vi "Get PublicEventRegistration.vi"(8 "error in (no error)":errorcluster, 11 "SMO":refnum<class "SMO.lvclass">) -> (0 "error out":errorcluster, 2 "SMO Public Events":refnum<event-registration>, 3 "SMO out":refnum<class "SMO.lvclass">)   [LabVIEW 2021, in "smo.lvlib" / "SMO.lvclass"]
doc: "This method has been deprecated. To achieve the same result, you should use the GetPublicEvents method and register for the events in the process."
uses:
  SMO.lvclass
  SMO.lvclass/SMO.ctl
  Typedefs/Public Events.ctl
  Typedefs/SMOState --Enum.ctl
  Typedefs/Reserve State--Enum.ctl
panel:
  # "For instructions on how to use the JKI State Machine Objects, examples and video tutorials, visit:\nhttp://jki.net/state-machine-objects/\n\nJKI State Machine Objects™\nhttp://jki.net/state-machine-objects/\nCopyright (C) 2005-2015, JKI <info@jki.net>\nALL RIGHTS RESERVED"
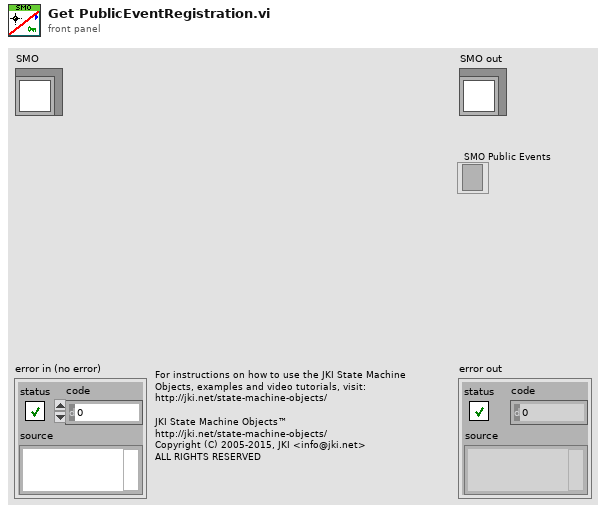
[diagram p1: front panel]
types:
  T1 = typedef "smo.lvlib/SMO.lvclass/Public Events.ctl" = cluster{"Error":refnum<user-event>, "State":refnum<user-event>, "Reserve State":refnum<user-event>}
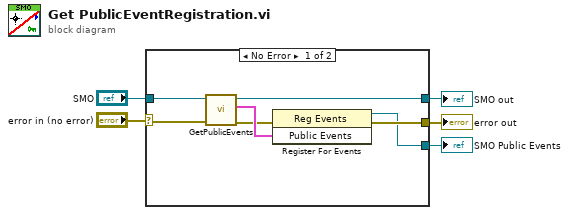
[diagram p0: block diagram]
diagram:
  n1 = case shown="No Error" "error in (no error)" {
    selector: "error in (no error)" -> [w7 w14]
    tunnel: [w12 w14] -> w2
    tunnel: [w8 w13] -> w3
    tunnel: "SMO" -> [w10 w13]
    tunnel: [w11 _] -> w1
    frame No Error {
      n2 = call "GetPublicEvents.vi"("error in (no error)"=w7, "SMO"=w10) -> ("error out"=w6:errorcluster, "Public Events"=w9:T1, "SMO out"=w8:refnum<class "SMO.lvclass">)  [unwired: 7 in]
      n3 = register-events(error in=w6, w9) -> (reference out=w11:refnum<event-registration>, error out=w12:errorcluster)  [unwired: 1 in]
    }
    frame Error {
    }
  }
  "error out" <- w2
  "SMO out" <- w3
  "SMO Public Events" <- w1
